vi "Hardware-KnockSetupCalPoints.vi"() -> (4 "Knock Settings":T2={"Low Cutoff [Hz]"=5000.0, "High Cutoff [Hz]"=6000.0, "Threshold"=2.0} {"High Cutoff [Hz]" format="%#_6p"; "Low Cutoff [Hz]" format="%#_6p"}, 6 "Knock Windows":T1={"Knock Start [CAD]"=0.0, "Knock End [CAD]"=20.0, "Reference Start [CAD]"=-70.0, "Reference End [CAD]"=-90.0}, 8 "Knock Sensor":i32[](array[ring]) items=["Sensor 1", "Sensor 2", "Sensor 3", "Sensor 4", "Sensor 5", "Sensor 6", "Sensor 7", "Sensor 8", "Sensor 9", "Sensor 10", "Sensor 11", "Sensor 12"], 10 "Knock Offset [CAD]":sgl[](array[numeric]))   [LabVIEW 2016, in "DSI-RT.lvlib"]
uses:
  DSI-RT.lvlib
  <vilib>/Powertrain Controls/Device Drivers/DCM/Tools/RT/Knock Settings.ctl
  <vilib>/Powertrain Controls/Device Drivers/FPGA Knock/RevA/RT/Controls/Windows.ctl
  <vilib>/addons/Software Calibration Management/xSCM/CalPoint.xnode
  <vilib>/Powertrain Controls/Device Drivers/DCM/Tools/RT/DCM - RT - Tools.lvlib
  <vilib>/Powertrain Controls/Device Drivers/FPGA Knock/RevA/RT/Knock - RevA - RT.lvlib
  <vilib>/addons/Software Calibration Management/xSCM/ni_scm.dll
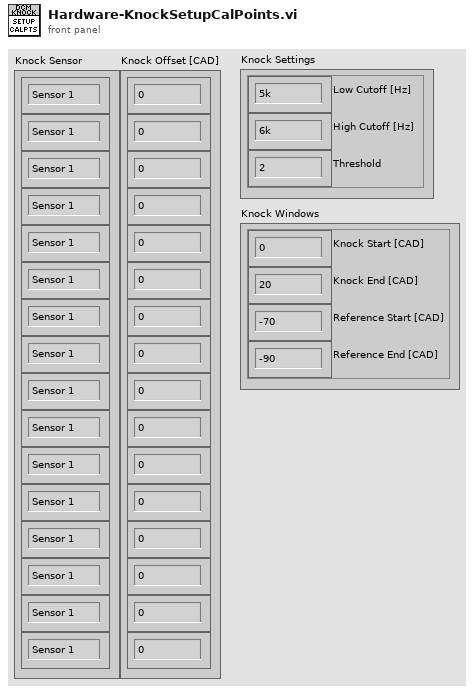
[diagram p1: front panel]
types:
  T1 = typedef "Knock - RevA - RT.lvlib/Windows.ctl" = cluster{"Knock Start [CAD]":sgl, "Knock End [CAD]":sgl, "Reference Start [CAD]":sgl, "Reference End [CAD]":sgl}
  T2 = typedef "DCM - RT - Tools.lvlib/Knock Settings.ctl" = cluster{"Low Cutoff [Hz]":sgl, "High Cutoff [Hz]":sgl, "Threshold":sgl}
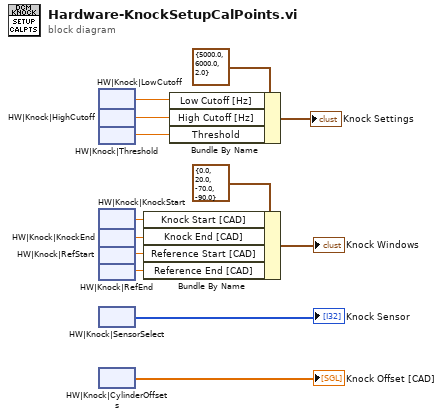
[diagram p0: block diagram]
diagram:
  n1 = xnode "HW|Knock|LowCutoff"() -> ("Value"=w13:sgl)
  n2 = xnode "HW|Knock|HighCutoff"() -> ("Value"=w12:sgl)
  n3 = xnode "HW|Knock|Threshold"() -> ("Value"=w11:sgl)
  n4 = xnode "HW|Knock|KnockStart"() -> ("Value"=w10:sgl)
  n5 = xnode "HW|Knock|KnockEnd"() -> ("Value"=w8:sgl)
  n6 = xnode "HW|Knock|RefStart"() -> ("Value"=w7:sgl)
  n7 = xnode "HW|Knock|RefEnd"() -> ("Value"=w9:sgl)
  n8 = xnode "HW|Knock|SensorSelect"() -> ("Value"=→"Knock Sensor":i32[])
  n9 = xnode "HW|Knock|CylinderOffsets"() -> ("Value"=→"Knock Offset [CAD]":sgl[])
  n10 = Bundle By Name(cluster=T1 {"Knock Start [CAD]"=0.0, "Knock End [CAD]"=20.0, "Reference Start [CAD]"=-70.0, "Reference End [CAD]"=-90.0} ("Knock Windows 2"), "Knock Start [CAD]"=w10, "Knock End [CAD]"=w8, "Reference Start [CAD]"=w7, "Reference End [CAD]"=w9) -> (→"Knock Windows":T1)
  n11 = Bundle By Name(cluster=T2 {"Low Cutoff [Hz]"=5000.0, "High Cutoff [Hz]"=6000.0, "Threshold"=2.0} ("Knock Settings 2"), "Low Cutoff [Hz]"=w13, "High Cutoff [Hz]"=w12, "Threshold"=w11) -> (→"Knock Settings":T2)
